vi "delete folder.vi"(8 "error in":errorcluster, 9 "folder":string, 10 "lib path":path, 11 "project in":refnum<vi>) -> (0 "error out":errorcluster, 3 "project out":refnum<vi>)   [LabVIEW 2014, in "SequencerActionScript.lvclass"]
doc: "NI Tag Bus Module Framework 1.0.2.36\nNI Systems Engineering"
uses:
  SequencerActionScript.lvclass
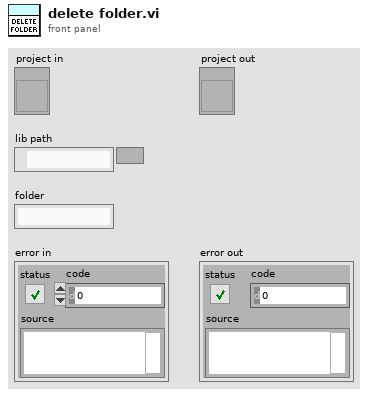
[diagram p1: front panel]
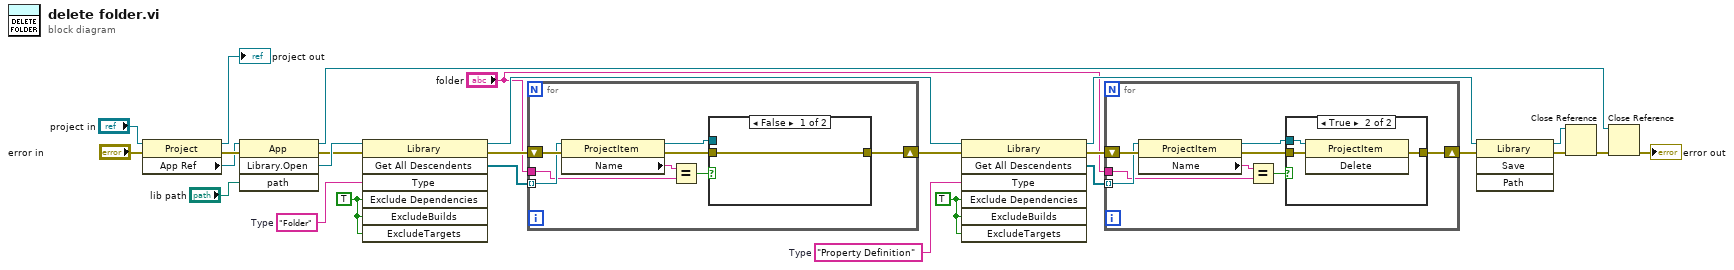
[diagram p0: block diagram]
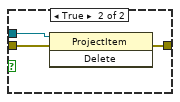
[diagram p3: hidden frame]
diagram:
  w9 = TRUE
  w6 = "Property Definition"  # Type
  w17 = TRUE
  w16 = "Folder"  # Type
  n1 = property class="Project"(reference="project in", error in="error in") -> (reference out=→"project out":refnum<vi>, error out=w13:errorcluster, "App Ref"=w12:refnum<vi>)
  n2 = invoke class="App" method="Library.Open"(reference=w12, error in=w13, "path"="lib path") -> (reference out=w24:refnum<vi>, error out=w18:errorcluster, "Open Library"=w19:refnum<vi>)  [unwired: 1 in, 1 out]
  n3 = invoke class="Library" method="Get All Descendents"(reference=w19, error in=w18, "Type"=w16, "Exclude Dependencies"=w17, "ExcludeBuilds"=w17, "ExcludeTargets"=w17) -> (reference out=w8:refnum<vi>, error out=w21:errorcluster, "All Descendents"=w20:refnum<vi>[])  [unwired: 1 in, 4 out]
  n4 = for {
    tunnel: w20 -> [w33] mode=indexing
    shift-right: [w28] -> w5
    shift-left: w21 -> [w34]
    tunnel: "folder" -> [w32]
    n5 = property class="ProjectItem"(reference=w33, error in=w34) -> (reference out=w30:refnum<vi>, error out=w29:errorcluster, "Name"=w31:string)
    n6 = Equal?(x=w31, y=w32) -> (x = y?=w27:bool)
    n7 = case shown="False" w27 {
      tunnel: w30 -> [_ w38]
      tunnel: w29 -> [w35 w37]
      tunnel: [w35 w36] -> w28
      frame False {
      }
      frame True {
        n8 = invoke class="ProjectItem" method="Delete"(reference=w38, error in=w37) -> (error out=w36:errorcluster)  [unwired: 1 in, 2 out]
      }
    }
  }
  n9 = invoke class="Library" method="Get All Descendents"(reference=w8, error in=w5, "Type"=w6, "Exclude Dependencies"=w9, "ExcludeBuilds"=w9, "ExcludeTargets"=w9) -> (reference out=w7:refnum<vi>, error out=w4:errorcluster, "All Descendents"=w3:refnum<vi>[])  [unwired: 1 in, 4 out]
  n10 = for {
    tunnel: w3 -> [w45] mode=indexing
    shift-right: [w40] -> w1
    shift-left: w4 -> [w46]
    tunnel: "folder" -> [w44]
    n11 = property class="ProjectItem"(reference=w45, error in=w46) -> (reference out=w42:refnum<vi>, error out=w41:errorcluster, "Name"=w43:string)
    n12 = Equal?(x=w43, y=w44) -> (x = y?=w39:bool)
    n13 = case shown="True" w39 {
      tunnel: w42 -> [_ w50]
      tunnel: w41 -> [w47 w49]
      tunnel: [w47 w48] -> w40
      frame False {
      }
      frame True {
        n14 = invoke class="ProjectItem" method="Delete"(reference=w50, error in=w49) -> (error out=w48:errorcluster)  [unwired: 1 in, 2 out]
      }
    }
  }
  n15 = invoke class="Library" method="Save"(reference=w7, error in=w1) -> (reference out=w23:refnum<vi>, error out=w22:errorcluster)  [unwired: 2 in, 2 out]
  n16 = Close Reference(reference=w23, error in (no error)=w22) -> (error out=w25:errorcluster)
  n17 = Close Reference(reference=w24, error in (no error)=w25) -> (error out=→"error out":errorcluster)
